vi "CmdExe.Launch Executable with Timeout, Abort, and Error Checks.vi"(4 "StdIn":string, 5 "Cmd IN Ref":refnum<vi>, 6 "Setup":T1={"Timeout (s)"=60.0, "Show Cmd Win"=FALSE, "Error Check"={"StdOut_Ck"=FALSE, "StdOutErrMsgs"=["Error", "Unable to find device "], "StdErr_Ck"=FALSE, "RtnCode_Ck"=FALSE, "RtnCodePASS"=0}, "Log_En"=FALSE, "LogFileName"="", "LogDir"=path ""}, 7 "Output Ref":refnum<vi>, 8 "error in (no error)":errorcluster, 9 "Ignore StdErr":bool, 10 "Args":string, 11 "Executable":path=path "C:/MTE/FW Load and Display Cal/Config/Bin/utahev_0_7/lighthouse_configtool.exe") -> (0 "error out":errorcluster, 1 "Duration(s)":dbl, 2 "return code":i32, 3 "Data Out":string)   [LabVIEW 2024]
uses:
  CmdExe.Setup Params.ctl
  CmdExe.Output Error Check Setup.ctl
  Errors/Error.Error Code List.ctl
  Errors.lvlib
  <vilib>/KATE/Time/Time Utils.lvlib
  <vilib>/KATE/Files/File Utils.lvlib
panel:
  out "Cmd":string
  out "Done":bool
  # "Launch Exe"
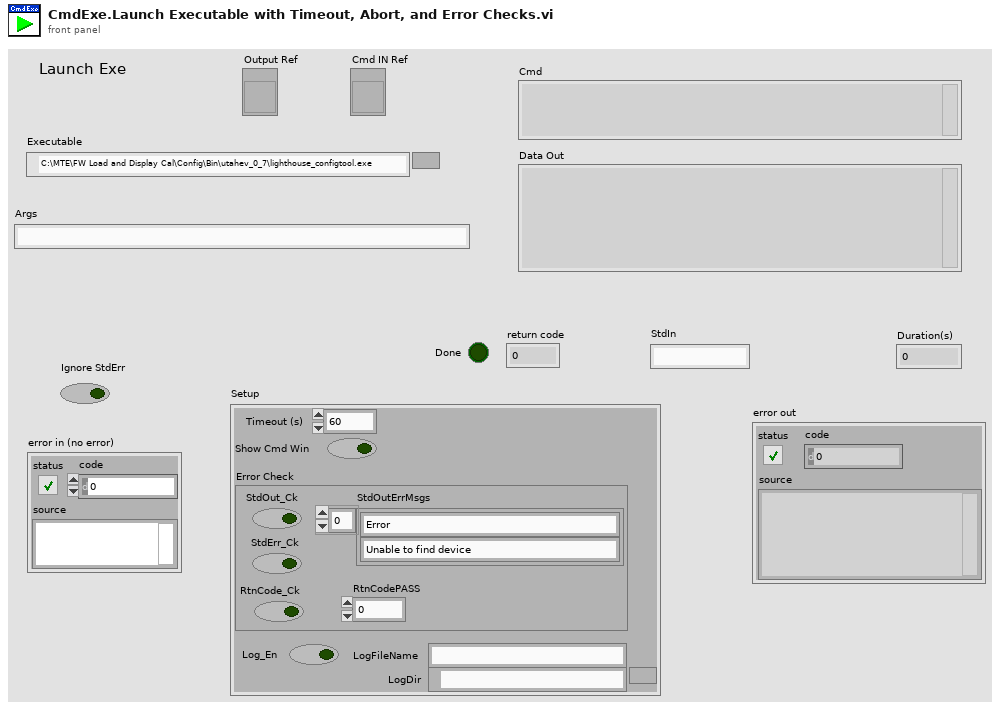
[diagram p1: front panel]
types:
  T1 = typedef "CmdExe.Setup Params.ctl" = cluster{"Timeout (s)":dbl, "Show Cmd Win":bool, "Error Check":T2, "Log_En":bool, "LogFileName":string, "LogDir":path}
  T2 = typedef "CmdExe.Output Error Check Setup.ctl" = cluster{"StdOut_Ck":bool, "StdOutErrMsgs":string[], "StdErr_Ck":bool, "RtnCode_Ck":bool, "RtnCodePASS":i32}
  T3 = enum16{"open", "replace", "create", "open or create", "replace or create", "replace or create with confirmation"}
  T4 = cluster{"Exe":string, "StdOut":string, "StdError":string, "LogFile":path, "Args":string, "TimedOut":bool, "RtnCode":i32, "LogEn":bool}
  T5 = typedef "EQMF.lvlib/Errors.lvlib/Error.Error Code List.ctl" = i32
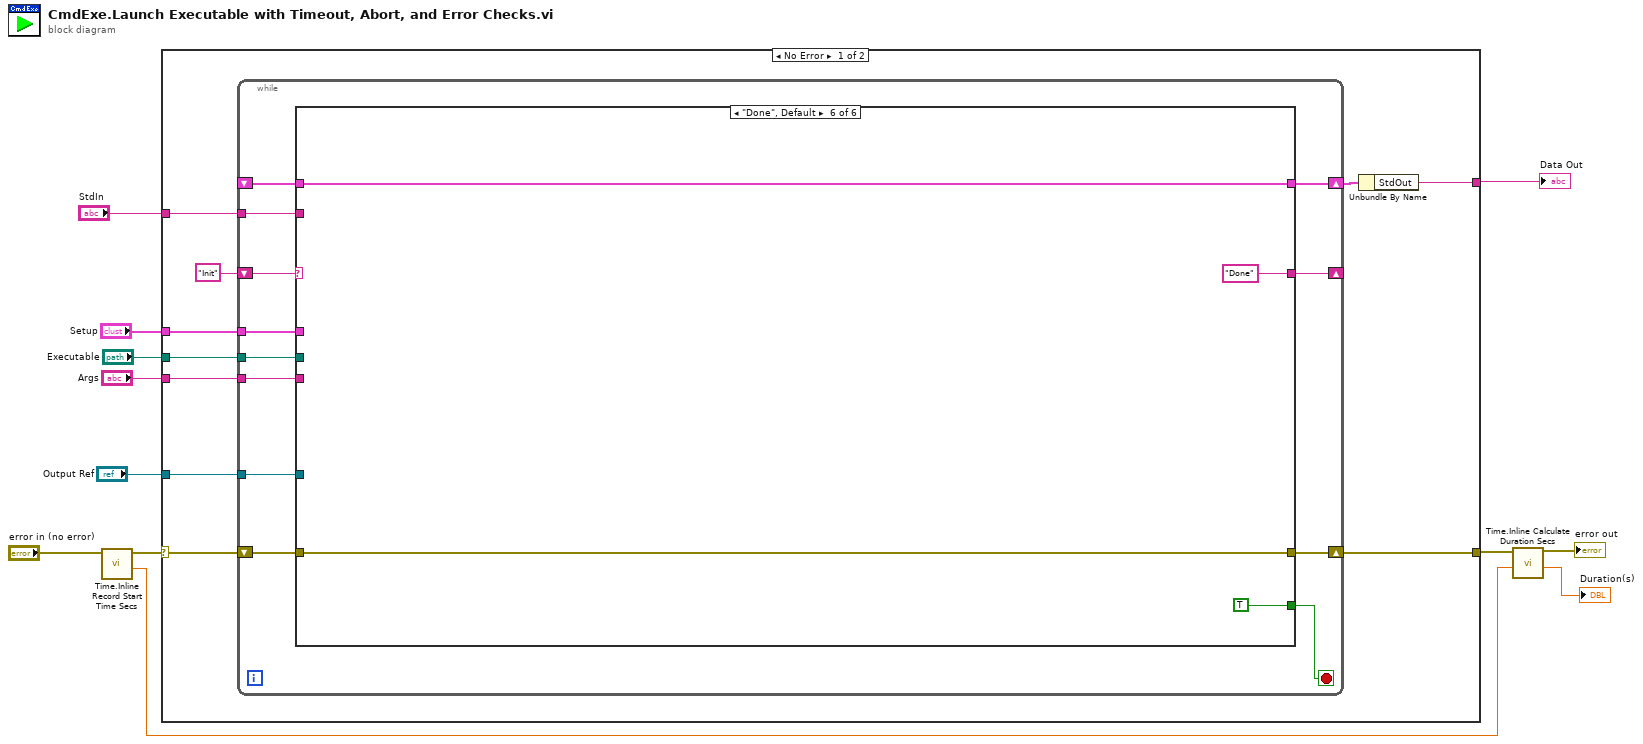
[diagram p0: block diagram]
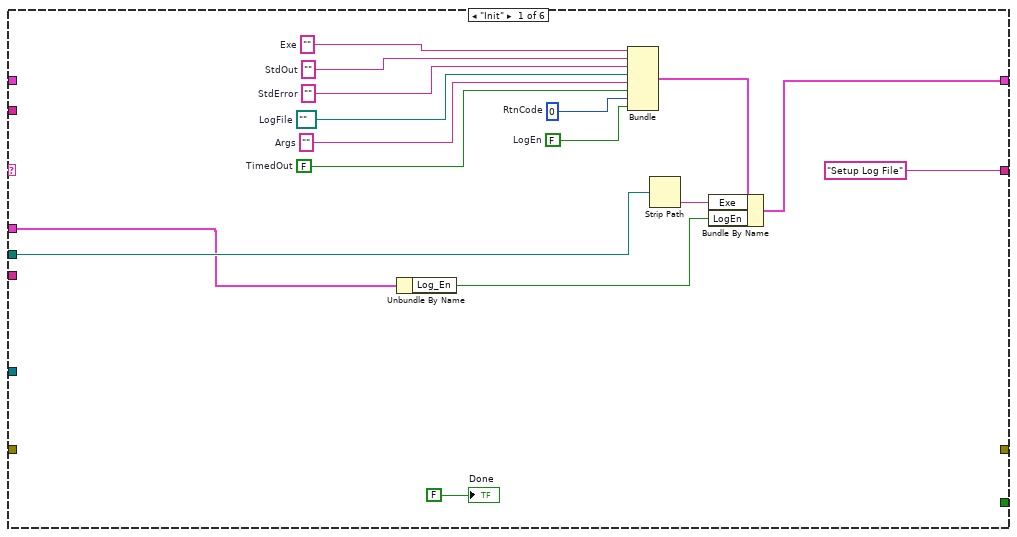
[diagram p2: hidden frame]
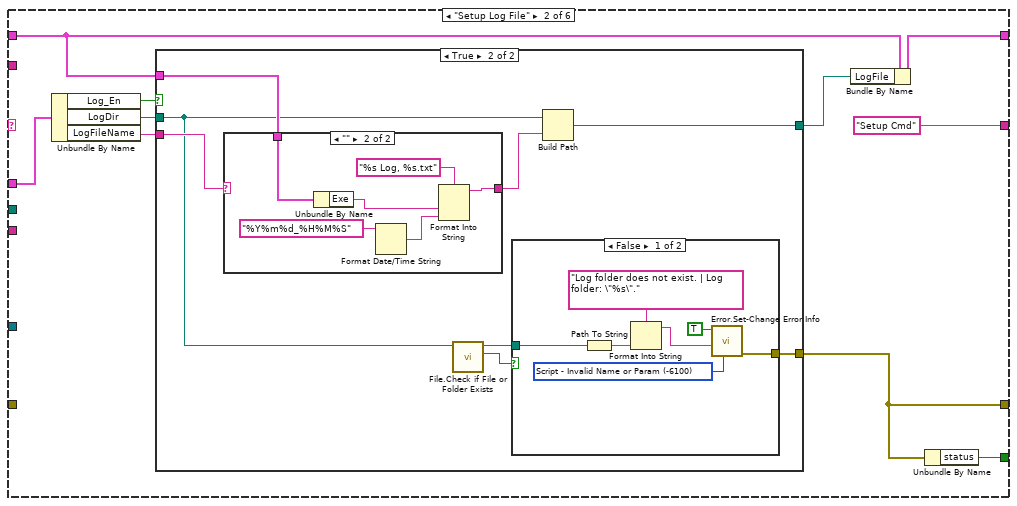
[diagram p3: hidden frame]
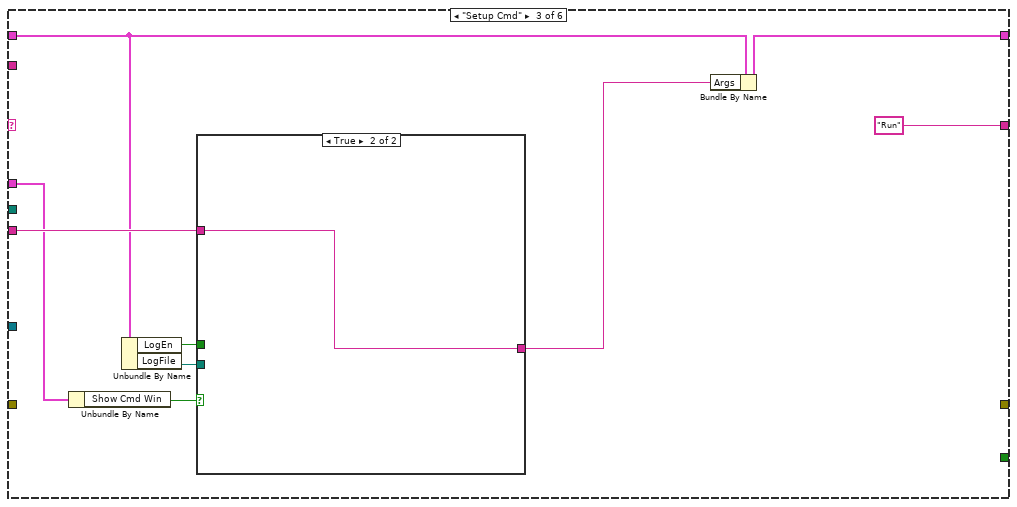
[diagram p7: hidden frame]
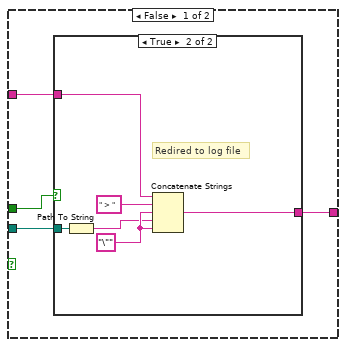
[diagram p8: hidden frame]
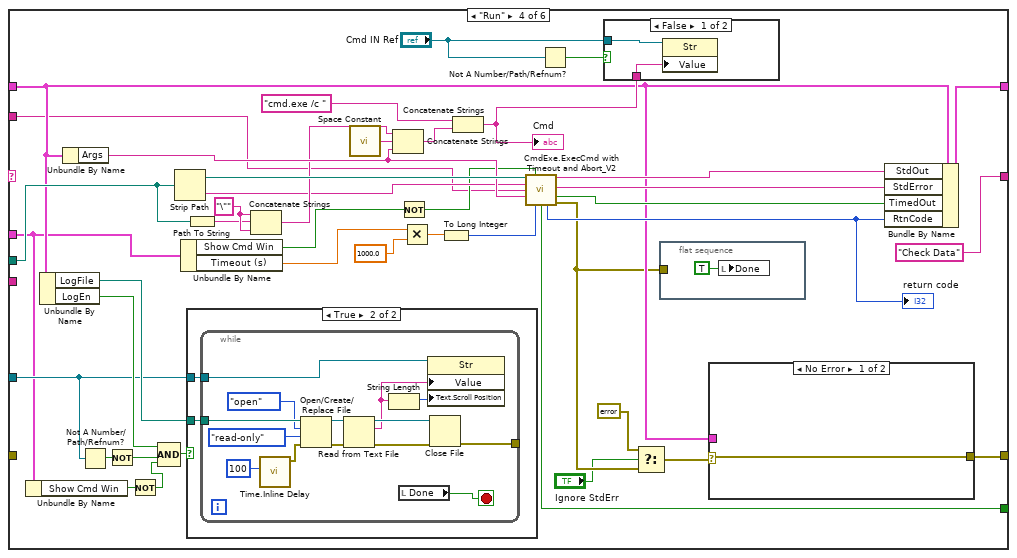
[diagram p10: hidden frame]
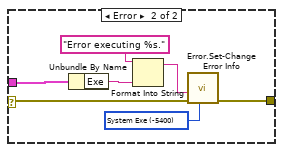
[diagram p11: hidden frame]
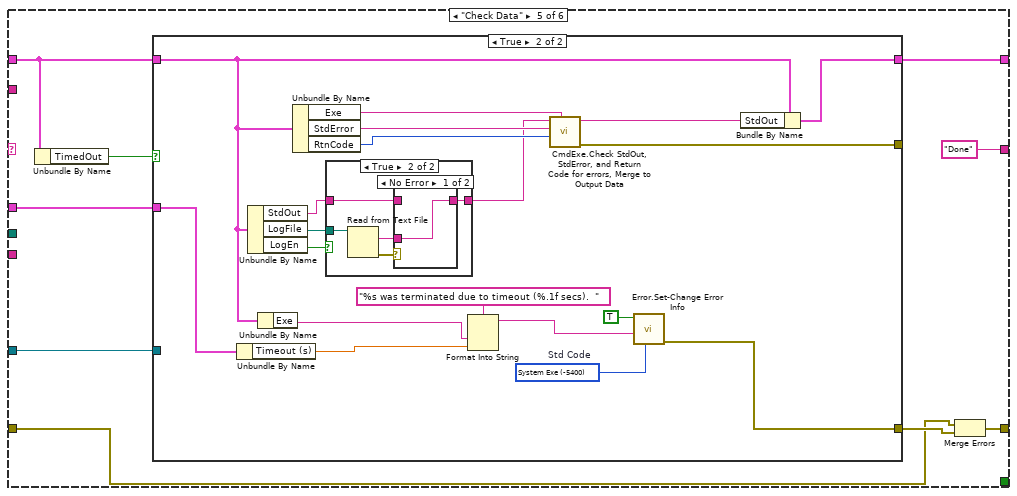
[diagram p14: hidden frame]
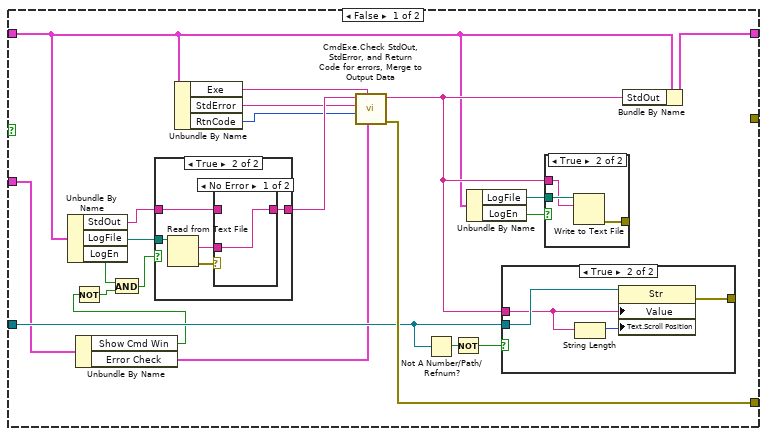
[diagram p15: hidden frame]
diagram:
  n1 = call <vilib>:"Time.Inline Record Start Time Secs.vi"("Error In Upper"="error in (no error)") -> ("Start(s)"=w9:dbl, "Error Out Upper"=w12:errorcluster)  [unwired: 8 in, 1 out]
  n2 = case shown="No Error" w12 {
    selector: w12 -> [w21 w249]
    tunnel: [w20 w249] -> w11
    tunnel: [w18 _] -> w10
    tunnel: "Executable" -> [w17 _]
    tunnel: "Args" -> [w16 _]
    tunnel: "Setup" -> [w15 _]
    tunnel: "Output Ref" -> [w14 _]
    tunnel: "StdIn" -> [w13 _]
    frame No Error {
      n3 = while {
        shift-right: [w32] -> w19
        shift-left: _ -> [w31]
        shift-right: [w24] -> _
        shift-left: "Init" -> [w34]
        shift-right: [w30] -> w20
        shift-left: w21 -> [w33]
        tunnel: w17 -> [w28]
        tunnel: w16 -> [w27]
        tunnel: w15 -> [w26]
        tunnel: w14 -> [w25]
        tunnel: w13 -> [w23]
        stop <- w29 stop-if-true
        n4 = case shown="\"Done\", Default" w34 {
          tunnel: ["Setup Log File" "Setup Cmd" "Run" "Check Data" "Done" "Done"] -> w24
          tunnel: w33 -> [_ _ _ _ w173 w245]
          tunnel: [w39 w59 w90 w145 w181 w246] -> w32
          tunnel: [_ w52 _ w113 w175 w245] -> w30
          tunnel: w31 -> [_ w57 w85 w112 w179 w246]
          tunnel: [_ w51 _ w141 _ TRUE] -> w29
          tunnel: w28 -> [w42 _ _ w126 _ _]
          tunnel: w27 -> [_ _ w88 _ _ _]
          tunnel: w26 -> [w36 w56 w84 w107 w177 _]
          tunnel: w25 -> [_ _ _ w114 w180 _]
          tunnel: w23 -> [_ _ _ w104 _ _]
          frame "Init" {
            w37 = FALSE  # LogEn
            w38 = 0  # RtnCode
            w43 = FALSE  # TimedOut
            w44 = ""  # Args
            w45 = path ""  # LogFile
            w46 = ""  # StdError
            w47 = ""  # StdOut
            w49 = ""  # Exe
            n5 = Unbundle By Name(w36) -> ("Log_En"=w35:bool)
            n6 = Bundle("Exe"=w49, "StdOut"=w47, "StdError"=w46, "LogFile"=w45, "Args"=w44, "TimedOut"=w43, "RtnCode"=w38, "LogEn"=w37) -> (w40:T4)  [unwired: 1 in]
            n7 = Strip Path(path=w42) -> (name=w41:string)  [unwired: 1 out]
            n8 = Bundle By Name(cluster=w40, "Exe"=w41, "LogEn"=w35) -> (w39:T4)
            "Done" <- FALSE ("Done")
          }
          frame "Setup Log File" {
            n9 = Unbundle By Name(w56) -> ("Log_En"=w55:bool, "LogDir"=w54:path, "LogFileName"=w53:string)
            n10 = case shown="True" w55 {
              tunnel: [_ w68] -> w58
              tunnel: w57 -> [_ w66]
              tunnel: w54 -> [_ w62]
              tunnel: w53 -> [_ w65]
              tunnel: [_ w61] -> w52
              frame False {
              }
              frame True {
                n11 = case shown="\"\"" w65 {
                  selector: w65 -> [w76 _]
                  tunnel: [w76 w79] -> w67
                  tunnel: w66 -> [_ w78]
                  frame Default {
                  }
                  frame "" {
                    n12 = Unbundle By Name(w78) -> ("Exe"=w77:string)
                    n13 = Format Date/Time String(time format string (%c)="%Y%m%d_%H%M%S") -> (date/time string=w82:string)  [unwired: 2 in]
                    n14 = Format Into String(format string="%s Log, %s.txt", w77, w82) -> (resulting string=w79:string)  [unwired: 2 in, 1 out]
                  }
                }
                n15 = call <vilib>:"File.Check if File or Folder Exists.vi"("Path"=w62) -> ("Exists"=w63:bool, "Dup Path"=w64:path)  [unwired: 6 in, 3 out]
                n16 = case shown="False" w63 {
                  tunnel: [w69 _] -> w61
                  tunnel: w64 -> [w73 _]
                  frame False {
                    w71 = T5 -6100 items=["No Error"=0, "Abort"=-2, "Misc"=-5000, "Fixture Error"=-5100, "File IO - General"=-5200, "FIle IO - Config Error"=-5201, "Instrument - General"=-5300, "Instrument - Serial Com"=-5301, "Instrument - Camera"=-5302, "Instrument - PS"=-5303, "Instrument - Oscilloscope"=-5304, "Instrument - Function Gen"=-5305, "Instrument - Load"=-5306, "Instrument - Meter"=-5307, "Instrument - Power Control"=-5308, "Instrument - Motion"=-5309, "Instrument - RF"=-5310, "System Exe"=-5400, "Image Processing"=-5500, "Communication"=-5600, "Script - Syntax Error"=-6000, "Script - Invalid Name or Param"=-6100, "Script - Timeout"=-6200, "Invalid Data"=-6300] ("Std Code")
                    n17 = Path To String(path=w73) -> (string=w74:string)
                    n18 = Format Into String(format string="Log folder does not exist. | Log folder: \"%s\".", w74) -> (resulting string=w70:string)  [unwired: 2 in, 1 out]
                    n19 = call "Error.Set-Change Error Info.vi"("Std Code"=w71, "Description"=w70, "Set Error"=TRUE) -> ("error out"=w69:errorcluster)  [unwired: 8 in]
                  }
                  frame True {
                    # "Folders exist.\nNo error."
                  }
                }
                n20 = Build Path(base path=w62, name or relative path=w67) -> (appended path=w68:path)
              }
            }
            n21 = Bundle By Name(cluster=w57, "LogFile"=w58) -> (w59:T4)
            n22 = Unbundle By Name(w52) -> ("status"=w51:bool)
          }
          frame "Setup Cmd" {
            n23 = Unbundle By Name(w84) -> ("Show Cmd Win"=w83:bool)
            n24 = Unbundle By Name(w85) -> ("LogEn"=w86:bool, "LogFile"=w89:path)
            n25 = case shown="True" w83 {
              tunnel: w89 -> [w95 _]
              tunnel: w88 -> [w94 w103]
              tunnel: [w93 w103] -> w87
              tunnel: w86 -> [w92 _]
              frame False {
                n26 = case shown="True" w92 {
                  tunnel: w95 -> [_ w99]
                  tunnel: w94 -> [w96 w98]
                  tunnel: [w96 w97] -> w93
                  frame False {
                  }
                  frame True {
                    w102 = "\""
                    # "Redired to log file"
                    n27 = Path To String(path=w99) -> (string=w101:string)
                    n28 = Concatenate Strings(w98, " > ", w102, w101, w102) -> (w97:string)
                  }
                }
              }
              frame True {
              }
            }
            n29 = Bundle By Name(cluster=w85, "Args"=w87) -> (w90:T4)
          }
          frame "Run" {
            w127 = "\""
            n30 = Unbundle By Name(w107) -> ("Show Cmd Win"=w106:bool)
            n31 = Unbundle By Name(w112) -> ("LogFile"=w135:path, "LogEn"=w119:bool)
            n32 = Unbundle By Name(w112) -> ("Args"=w128:string)
            n33 = Not A Number/Path/Refnum?(number/path/refnum=w114) -> (NaN/Path/Refnum?=w122:bool)
            n34 = Not(x=w122) -> (.not. x?=w121:bool)
            n35 = Not(x=w106) -> (.not. x?=w105:bool)
            n36 = Compound Arithmetic op=AND(w119, w121, w105) -> (w120:bool)
            n37 = Strip Path(path=w126) -> (stripped path=w134:path, name=w123:string)
            n38 = Unbundle By Name(w107) -> ("Show Cmd Win"=w117:bool, "Timeout (s)"=w118:dbl)
            n39 = Path To String(path=w126) -> (string=w125:string)
            n40 = case shown="True" w120 {
              tunnel: w135 -> [_ w157]
              tunnel: w114 -> [_ w158]
              frame False {
              }
              frame True {
                n41 = while {
                  tunnel: w158 -> [w164]
                  tunnel: w157 -> [w168]
                  tunnel: [w167] -> _
                  stop <- w163 stop-if-true
                  n42 = call <vilib>:"Time.Inline Delay.vi"("Wait(ms)"=u32 100) -> ("error out top"=w161:errorcluster)  [unwired: 9 in, 1 out]
                  n43 = Open/Create/Replace File(file path (use dialog)=w168, error in=w161, operation (0:open)=T3."open", access (0:read/write)=enum16{"read/write", "read-only", "write-only"}."read-only") -> (refnum out=w169:refnum<file>, error out=w172:errorcluster)  [unwired: 2 in, 1 out]
                  n44 = Read from Text File(file (use dialog)=w169, error in=w172) -> (refnum out=w170:refnum<file>, text=w160:string, error out=w171:errorcluster)  [unwired: 2 in, 1 out]
                  n45 = String Length(string=w160) -> (length=w159:i32)
                  n46 = local read "Done"() -> (w163:bool)
                  n47 = property class="Str"(reference=w164, "Value"=w160, "Text.Scroll Position"=w159) -> ()  [unwired: 1 in, 2 out]
                  n48 = Close File(refnum=w170, error in=w171) -> (error out=w167:errorcluster)  [unwired: 1 out]
                }
              }
            }
            n49 = Concatenate Strings(w127, w125, w127) -> (w124:string)
            n50 = call <vilib>:"Space Constant.vi"() -> ("String"=w131:string)
            n51 = Concatenate Strings(w124, w131, w128) -> (w132:string)
            n52 = Not(x=w117) -> (.not. x?=w116:bool)
            n53 = Multiply(x=w118, y=1000.0) -> (x*y=w140:dbl)
            n54 = To Long Integer(number=w140) -> (32bit integer=w138:i32)
            n55 = Concatenate Strings("cmd.exe /c ", w132) -> (w130:string)
            "Cmd" <- w130
            n56 = call "CmdExe.ExecCmd with Timeout and Abort_V2.vi"("Working Dir"=w134, "Run minimized? (T)"=w116, "Executable"=w123, "StdIn"=w104, "Arguements"=w128, "Timeout ms(-1)"=w138) -> ("STD OUT"=w115:string, "STD ERR"=w144:string, "Timed Out"=w143:bool, "Aborted"=w141:bool, "return code"=w129:i32, "error out"=w111:errorcluster)  [unwired: 4 in]
            "return code" <- w129
            n57 = Not A Number/Path/Refnum?(number/path/refnum="Cmd IN Ref") -> (NaN/Path/Refnum?=w137:bool)
            n58 = case shown="False" w137 {
              tunnel: "Cmd IN Ref" -> [w156 _]
              tunnel: w130 -> [w155 _]
              frame False {
                n59 = property class="Str"(reference=w156, "Value"=w155) -> ()  [unwired: 1 in, 2 out]
              }
              frame True {
              }
            }
            n60 = Select(t=errorcluster {"status"=FALSE, "code"=0, "source"=""}, s="Ignore StdErr", f=w111) -> (s? t:f=w110:errorcluster)
            n61 = flat-sequence {
              tunnel: w111 -> [_]
              frame #0 {
                n62 = local write "Done"(TRUE ("Done")) -> ()
              }
            }
            n63 = case shown="No Error" w110 {
              selector: w110 -> [w146 w149]
              tunnel: [w146 w148] -> w113
              tunnel: w112 -> [_ w147]
              frame No Error {
              }
              frame Error {
                w151 = T5 -5400 items=["No Error"=0, "Abort"=-2, "Misc"=-5000, "Fixture Error"=-5100, "File IO - General"=-5200, "FIle IO - Config Error"=-5201, "Instrument - General"=-5300, "Instrument - Serial Com"=-5301, "Instrument - Camera"=-5302, "Instrument - PS"=-5303, "Instrument - Oscilloscope"=-5304, "Instrument - Function Gen"=-5305, "Instrument - Load"=-5306, "Instrument - Meter"=-5307, "Instrument - Power Control"=-5308, "Instrument - Motion"=-5309, "Instrument - RF"=-5310, "System Exe"=-5400, "Image Processing"=-5500, "Communication"=-5600, "Script - Syntax Error"=-6000, "Script - Invalid Name or Param"=-6100, "Script - Timeout"=-6200, "Invalid Data"=-6300] ("Std Code")
                n64 = Unbundle By Name(w147) -> ("Exe"=w152:string)
                n65 = Format Into String(format string="Error executing %s.", w152) -> (resulting string=w150:string)  [unwired: 2 in, 1 out]
                n66 = call "Error.Set-Change Error Info.vi"("Std Code"=w151, "error in"=w149, "Description"=w150) -> ("error out"=w148:errorcluster)  [unwired: 8 in]
              }
            }
            n67 = Bundle By Name(cluster=w112, "StdOut"=w115, "StdError"=w144, "TimedOut"=w143, "RtnCode"=w129) -> (w145:T4)
          }
          frame "Check Data" {
            n68 = Unbundle By Name(w179) -> ("TimedOut"=w178:bool)
            n69 = case shown="True" w178 {
              tunnel: [w202 w224] -> w181
              tunnel: w179 -> [w186 w218]
              tunnel: [w197 w229] -> w174
              tunnel: w180 -> [w194 _]
              tunnel: w177 -> [w191 w234]
              tunnel: [_ w219] -> _
              frame False {
                n70 = Unbundle By Name(w186) -> ("StdOut"=w192:string, "LogFile"=w201:path, "LogEn"=w185:bool)
                n71 = Unbundle By Name(w191) -> ("Show Cmd Win"=w183:bool, "Error Check"=w190:T2)
                n72 = Not(x=w183) -> (.not. x?=w184:bool)
                n73 = And(x=w185, y=w184) -> (x .and. y?=w182:bool)
                n74 = case shown="True" w182 {
                  tunnel: w201 -> [_ w215]
                  tunnel: [w210 w213] -> w200
                  tunnel: w192 -> [w210 w211]
                  frame False {
                    (unwired) TRUE
                  }
                  frame True {
                    n75 = Read from Text File(file (use dialog)=w215) -> (text=w212:string, error out=w214:errorcluster)  [unwired: 3 in, 2 out]
                    n76 = case shown="No Error" w214 {
                      tunnel: [w216 w217] -> w213
                      tunnel: w212 -> [w216 _]
                      tunnel: w211 -> [_ w217]
                      frame No Error {
                      }
                      frame Error {
                      }
                    }
                  }
                }
                n77 = Unbundle By Name(w186) -> ("Exe"=w193:string, "StdError"=w199:string, "RtnCode"=w198:i32)
                n78 = call "CmdExe.Check StdOut, StdError, and Return Code for errors, Merge to Output Data.vi"("Error Check"=w190, "App Name"=w193, "Return Code"=w198, "StdError"=w199, "StdOut"=w200) -> ("error out"=w197:errorcluster, "Output Data"=w187:string)  [unwired: 5 in]
                n79 = Not A Number/Path/Refnum?(number/path/refnum=w194) -> (NaN/Path/Refnum?=w196:bool)
                n80 = Not(x=w196) -> (.not. x?=w195:bool)
                n81 = Unbundle By Name(w186) -> ("LogFile"=w189:path, "LogEn"=w188:bool)
                n82 = case shown="True" w195 {
                  tunnel: w194 -> [_ w208]
                  tunnel: w187 -> [_ w207]
                  tunnel: [_ w206] -> _
                  frame False {
                  }
                  frame True {
                    n83 = String Length(string=w207) -> (length=w209:i32)
                    n84 = property class="Str"(reference=w208, "Value"=w207, "Text.Scroll Position"=w209) -> (error out=w206:errorcluster)  [unwired: 1 in, 1 out]
                  }
                }
                n85 = case shown="True" w188 {
                  tunnel: w189 -> [_ w205]
                  tunnel: [_ w204] -> _
                  tunnel: w187 -> [_ w203]
                  frame False {
                    (unwired) TRUE
                  }
                  frame True {
                    n86 = Write to Text File(file (use dialog)=w205, text=w203) -> (error out=w204:errorcluster)  [unwired: 2 in, 2 out]
                  }
                }
                n87 = Bundle By Name(cluster=w186, "StdOut"=w187) -> (w202:T4)
              }
              frame True {
                w232 = T5 -5400 items=["No Error"=0, "Abort"=-2, "Misc"=-5000, "Fixture Error"=-5100, "File IO - General"=-5200, "FIle IO - Config Error"=-5201, "Instrument - General"=-5300, "Instrument - Serial Com"=-5301, "Instrument - Camera"=-5302, "Instrument - PS"=-5303, "Instrument - Oscilloscope"=-5304, "Instrument - Function Gen"=-5305, "Instrument - Load"=-5306, "Instrument - Meter"=-5307, "Instrument - Power Control"=-5308, "Instrument - Motion"=-5309, "Instrument - RF"=-5310, "System Exe"=-5400, "Image Processing"=-5500, "Communication"=-5600, "Script - Syntax Error"=-6000, "Script - Invalid Name or Param"=-6100, "Script - Timeout"=-6200, "Invalid Data"=-6300]  # Std Code
                n88 = Unbundle By Name(w234) -> ("Timeout (s)"=w233:dbl)
                n89 = Unbundle By Name(w218) -> ("StdOut"=w221:string, "LogFile"=w223:path, "LogEn"=w222:bool)
                n90 = Unbundle By Name(w218) -> ("Exe"=w235:string)
                n91 = Unbundle By Name(w218) -> ("Exe"=w226:string, "StdError"=w228:string, "RtnCode"=w227:i32)
                n92 = case shown="True" w222 {
                  tunnel: w223 -> [_ w242]
                  tunnel: [w237 w240] -> w220
                  tunnel: w221 -> [w237 w238]
                  frame False {
                    (unwired) TRUE
                  }
                  frame True {
                    n93 = Read from Text File(file (use dialog)=w242) -> (text=w239:string, error out=w241:errorcluster)  [unwired: 3 in, 2 out]
                    n94 = case shown="No Error" w241 {
                      tunnel: [w243 w244] -> w240
                      tunnel: w239 -> [w243 _]
                      tunnel: w238 -> [_ w244]
                      frame No Error {
                      }
                      frame Error {
                      }
                    }
                  }
                }
                n95 = Format Into String(format string="%s was terminated due to timeout (%.1f secs).  ", w235, w233) -> (resulting string=w230:string)  [unwired: 2 in, 1 out]
                n96 = call "CmdExe.Check StdOut, StdError, and Return Code for errors, Merge to Output Data.vi"("App Name"=w226, "Return Code"=w227, "StdError"=w228, "StdOut"=w220) -> ("error out"=w219:errorcluster, "Output Data"=w225:string)  [unwired: 6 in]
                n97 = call "Error.Set-Change Error Info.vi"("Std Code"=w232, "Description"=w230, "Set Error"=TRUE) -> ("error out"=w229:errorcluster)  [unwired: 8 in]
                n98 = Bundle By Name(cluster=w218, "StdOut"=w225) -> (w224:T4)
              }
            }
            n99 = Merge Errors(w173, w174) -> (w175:errorcluster)
          }
          frame "Done", Default {
          }
        }
      }
      n100 = Unbundle By Name(w19) -> ("StdOut"=w18:string)
    }
    frame Error {
    }
  }
  "Data Out" <- w10
  n101 = call <vilib>:"Time.Inline Calculate Duration Secs.vi"("Start(Sec)"=w9, "Error In Top"=w11) -> ("Duration(s)"=→"Duration(s)":dbl, "Error Out Top"=→"error out":errorcluster)  [unwired: 7 in, 1 out]
